vi "重测原因.vi"() -> (1 "重测原因str":string, 2 "继续":bool)   [LabVIEW 2011]
panel:
  in  "取消按钮":bool
  in  "确定按钮":bool
  in  "重测原因":T1(radio)
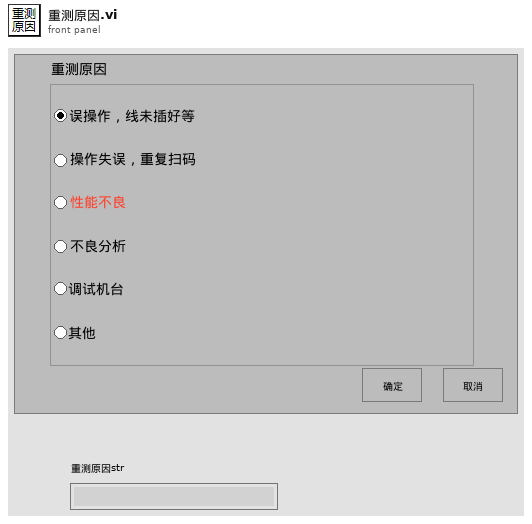
[diagram p1: front panel]
types:
  T1 = enum32{"误操作，线未插好等", "性能不良", "不良分析", "其他", "调试机台", "操作失误，重复扫码"}
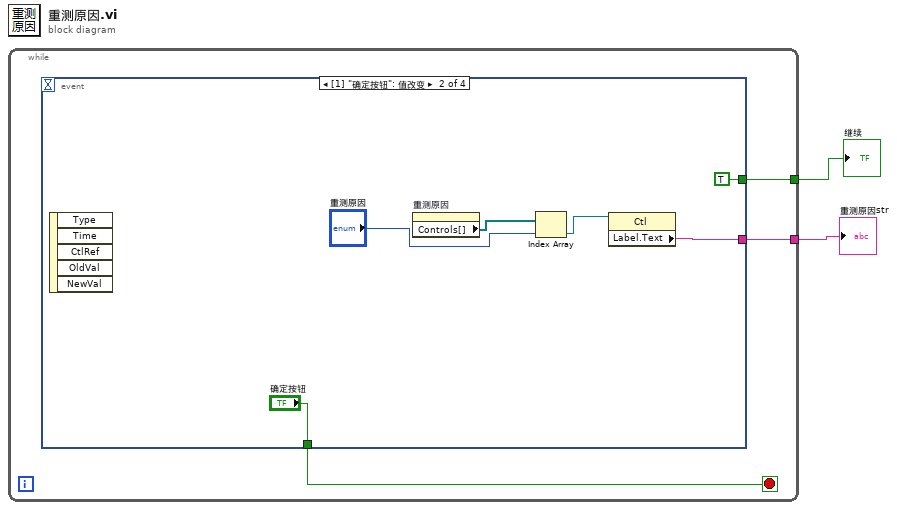
[diagram p0: block diagram]
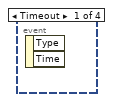
[diagram p2: hidden frame]
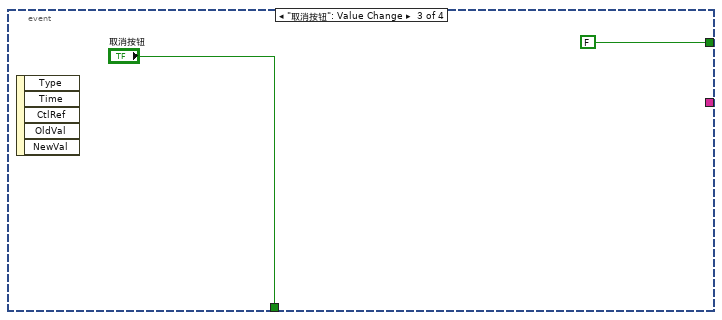
[diagram p3: hidden frame]
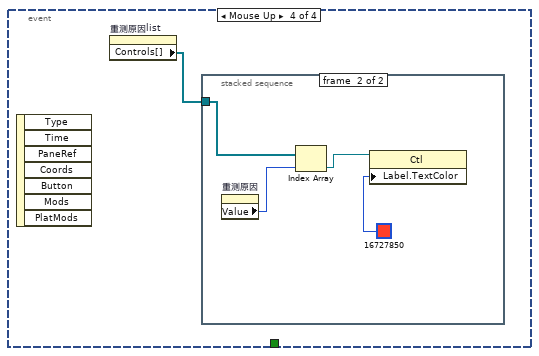
[diagram p4: hidden frame]
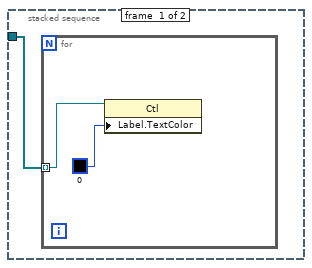
[diagram p5: hidden frame]
diagram:
  n1 = while {
    tunnel: [w4] -> w2
    tunnel: [w3] -> w1
    stop <- w5 stop-if-true
    n2 = event shown="[1] \"确定按钮\": 值改变" {
      selector: _ -> [_ _ _ _]
      dyn-events: _ -> [_ _ _ _]
      timeout: _ -> [_ _ _ _]
      tunnel: [_ "确定按钮" "取消按钮" _] -> w5
      tunnel: [_ w8 _ _] -> w4
      tunnel: [_ TRUE FALSE _] -> w3
      event Timeout {
        n3 = event-data() -> ()  [unwired: 1 in, 2 out]
      }
      event "确定按钮": Value Change {
        n4 = event-data() -> ()  [unwired: 1 in, 5 out]
        n5 = property on="重测原因" class="RadioBtnsControl (严格)"() -> ("Controls[]"=w10:refnum<vi>[])  [unwired: 2 in, 2 out]
        n6 = Index Array(array=w10, index="重测原因") -> (element=w9:refnum<vi>)
        n7 = property class="Ctl"(reference=w9) -> ("Label.Text"=w8:string)  [unwired: 1 in, 2 out]
      }
      event "取消按钮": Value Change {
        n8 = event-data() -> ()  [unwired: 1 in, 5 out]
      }
      event Mouse Up {
        n9 = event-data() -> ()  [unwired: 1 in, 7 out]
        n10 = property on="重测原因list" class="RadioBtnsControl (严格)"() -> ("Controls[]"=w14:refnum<vi>[])  [unwired: 2 in, 2 out]
        n11 = stacked-sequence {
          tunnel: w14 -> [w15 w20]
          frame #0 {
            n12 = for {
              tunnel: w15 -> [w17] mode=indexing
              n13 = property class="Ctl"(reference=w17, "Label.TextColor"=u32 0) -> ()  [unwired: 1 in, 2 out]
            }
          }
          frame #1 {
            n14 = property on="重测原因" class="RadioBtnsControl (严格)"() -> ("Value"=w19:T1)  [unwired: 2 in, 2 out]
            n15 = Index Array(array=w20, index=w19) -> (element=w18:refnum<vi>)
            n16 = property class="Ctl"(reference=w18, "Label.TextColor"=u32 16727850) -> ()  [unwired: 1 in, 2 out]
          }
        }
      }
    }
  }
  "重测原因str" <- w2
  "继续" <- w1
